vi "Complete Request.vi"(7 "Inputs":T2, 8 "error in (no error)":errorcluster, 11 "Session Cleanup Handler in":refnum<class "Session Cleanup Handler.lvclass">) -> (0 "error out":errorcluster, 5 "Outputs":T1)   [LabVIEW 2020, in "HTTP Server.lvlib" / "Session Cleanup Handler.lvclass"]
uses:
  Session Cleanup Handler.lvclass
  Cleanup Inputs.ctl
  Values/Values.lvclass
  <vilib>/IlluminatedG/IG HTTP Utils/HTTP Utils/Request/Request.lvclass
  <vilib>/IlluminatedG/IG HTTP Utils/HTTP Utils/Response/Response.lvclass
  Session/Session.lvclass
  Cleanup Outputs.ctl
  Session Cleanup Handler.lvclass/Session Cleanup Handler.ctl
  HTTP Server.lvlib
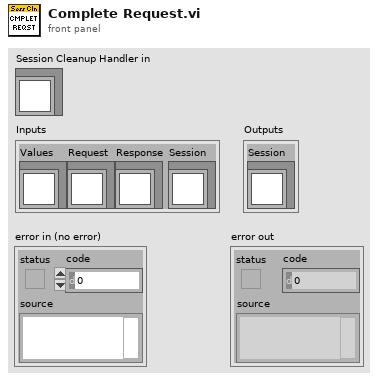
[diagram p1: front panel]
types:
  T1 = typedef "HTTP Server.lvlib/Cleanup Outputs.ctl" = cluster{"Session":refnum<class "Session.lvclass">}
  T2 = typedef "HTTP Server.lvlib/Cleanup Inputs.ctl" = cluster{"Values":refnum<class "Values.lvclass">, "Request":refnum<class "Request.lvclass">, "Response":refnum<class "Response.lvclass">, "Session":refnum<class "Session.lvclass">}
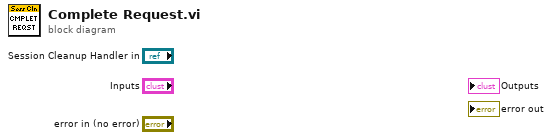
[diagram p0: block diagram]
diagram:
